vi "tes_format_sincos.vi"(8 "valid in":bool, 10 "cos_fi":fxp<+/-,16,2>, 11 "sin fi":fxp<+/-,16,2>) -> (0 "valid out":bool, 3 "Element":u64[](array[numeric]))   [LabVIEW 2013]
uses:
  <vilib>/rvi/FXPMathLib/FxpInterpret/XNode/nifxpmath_Interpret.xnode
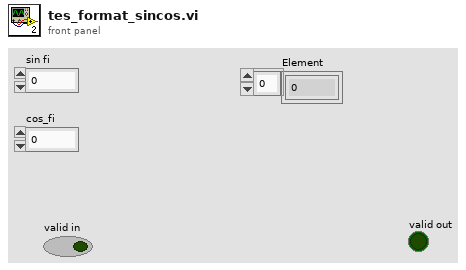
[diagram p1: front panel]
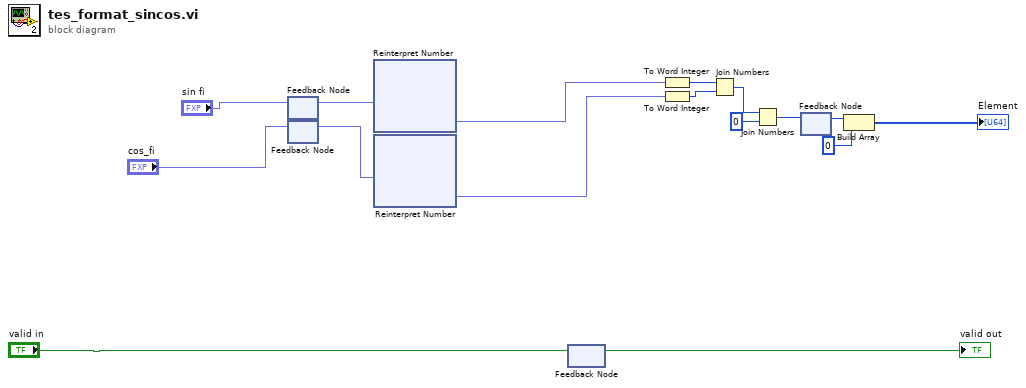
[diagram p0: block diagram]
diagram:
  n1 = feedback #1() -> (w12:fxp<+/-,16,2>)  [unwired: 1 in]
  n2 = feedback-in #1("sin fi") -> ()
  n3 = feedback #2() -> (w10:fxp<+/-,16,2>)  [unwired: 1 in]
  n4 = feedback-in #2("cos_fi") -> ()
  n5 = xnode "Reinterpret Number"("x"=w12) -> ("y"=w11:fxp<+/-,16,16>)
  n6 = xnode "Reinterpret Number"("x"=w10) -> ("y"=w9:fxp<+/-,16,16>)
  n7 = feedback #3() -> (→"valid out":bool)  [unwired: 1 in]
  n8 = feedback-in #3("valid in") -> ()
  n9 = To Word Integer(number=w11) -> (16bit integer=w14:i16)
  n10 = To Word Integer(number=w9) -> (16bit integer=w15:i16)
  n11 = Join Numbers(hi=w14, lo=w15) -> ((hi.lo)=w13:u32)
  n12 = Join Numbers(hi=w13, lo=u32 0) -> ((hi.lo)=w8:u64)
  n13 = feedback #4() -> (w7:u64)  [unwired: 1 in]
  n14 = feedback-in #4(w8) -> ()
  n15 = Build Array(w7, u64 0 ("element")) -> (→"Element":u64[])
